vi "Build Channel Cluster Array.vi"(11 "Channels Amount":u8) -> (3 "Channels out":cluster{"Channels":T1[]})   [LabVIEW 2023, in "Climate Chamber Cluster.lvclass"]
uses:
  Climate Chamber Cluster.lvclass
  Utilities/Channel.ctl
  Climate Chamber Cluster.lvclass/Climate Chamber Cluster.ctl
  Utilities/Utilities.lvlib
panel:
  in  "Climate Chamber Cluster.lvclass":refnum<class "Climate Chamber Cluster.lvclass">
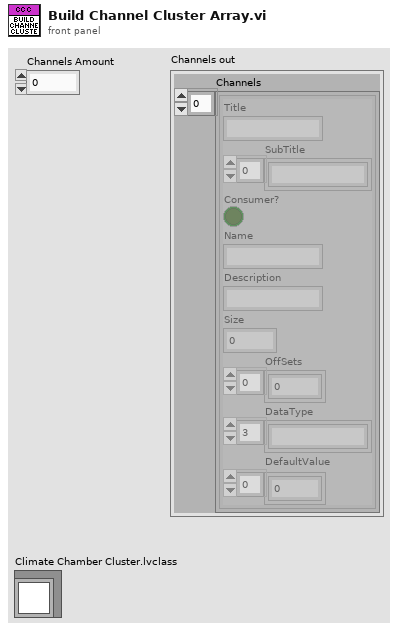
[diagram p1: front panel]
types:
  T1 = typedef "Utilities.lvlib/Channel.ctl" = cluster{"Title":string, "SubTitle":string[], "Consumer?":bool, "Name":string, "Description":string, "Size":i32, "OffSets":i32[], "DataType":string[], "DefaultValue":dbl[]}
  T2 = cluster{"OnOff.ACT":bool, "ErrorAcknowledge.ACT":bool}
  T3 = cluster{"OnOff.STS":i32, "Error.STS":i32, "Watchdog.STS":i32}
  T4 = cluster{"Temperature.SP":dbl, "TemperatureMIN.SP":dbl, "TemperatureMAX.SP":dbl, "TemperatureGrad.SP":dbl, "Humidity.SP":dbl, "HumidityMIN.SP":dbl, "HumidityMAX.SP":dbl, "HumidityGrad.SP":dbl}[]
  T5 = cluster{"Temperature.AV":dbl, "Humidity.AV":dbl}[]
  T6 = cluster{"Temperature.SP":dbl, "TemperatureMIN.SP":dbl, "TemperatureMAX.SP":dbl, "TemperatureGrad.SP":dbl, "Humidity.SP":dbl, "HumidityMIN.SP":dbl, "HumidityMAX.SP":dbl, "HumidityGrad.SP":dbl}
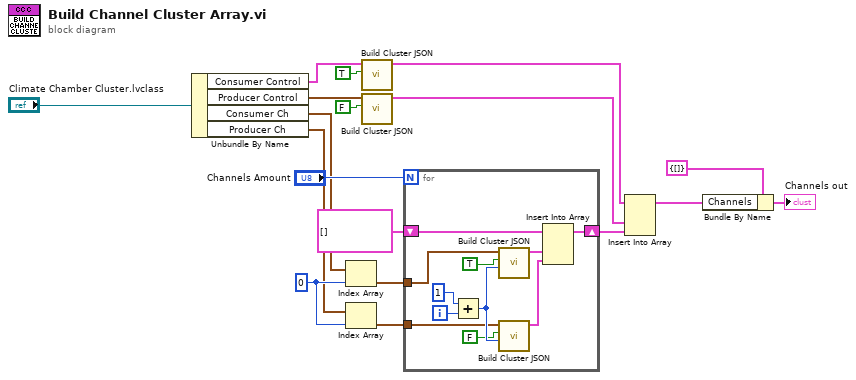
[diagram p0: block diagram]
diagram:
  w3 = 0 ("index")
  n1 = Unbundle By Name("Climate Chamber Cluster.lvclass") -> ("Consumer Control"=w8:T2, "Producer Control"=w7:T3, "Consumer Ch"=w5:T4, "Producer Ch"=w2:T5)
  n2 = Index Array(array=w5, index=w3) -> (element=w4:T6)
  n3 = Index Array(array=w2, index=w3) -> (element=w1:cluster{"Temperature.AV":dbl, "Humidity.AV":dbl})
  n4 = call "Build Cluster JSON.vi"("Consumer?"=TRUE, "Cluster"=w8) -> ("Array"=w15:T1[])  [unwired: 9 in]
  n5 = call "Build Cluster JSON.vi"("Consumer?"=FALSE, "Cluster"=w7) -> ("Array"=w14:T1[])  [unwired: 9 in]
  n6 = for {
    N: "Channels Amount" -> [_]
    shift-right: [w25] -> w12
    shift-left: T1[] [] -> [w26]
    tunnel: w4 -> [w21]
    tunnel: w1 -> [w19]
    i -> [w24]
    n7 = Add(x=1, y=w24) -> (x+y=w22:i32)
    n8 = call "Build Cluster JSON.vi"("Channels Amount"=w22, "Consumer?"=TRUE, "Cluster"=w21) -> ("Array"=w28:T1[])  [unwired: 8 in]
    n9 = call "Build Cluster JSON.vi"("Channels Amount"=w22, "Consumer?"=FALSE, "Cluster"=w19) -> ("Array"=w27:T1[])  [unwired: 8 in]
    n10 = Insert Into Array(array=w26, new element #1=w28, new element #2=w27) -> (w25:T1[])  [unwired: 1 in]
  }
  n11 = Insert Into Array(array=w15, new element #1=w14, new element #2=w12) -> (w10:T1[])  [unwired: 1 in]
  n12 = Bundle By Name(cluster=cluster{"Channels":T1[]} {"Channels"=[]} ("Channels in"), "Channels"=w10) -> (→"Channels out":cluster{"Channels":T1[]})
